vi "SetOverVoltProtLimit.vi"(8 "error in (no error)":errorcluster, 9 "Voltage":dbl, 11 "VISA resource name":refnum<visa-resource-name>) -> (0 "error out":errorcluster, 3 "VISA resource name out":refnum<visa-resource-name>)   [LabVIEW 2019, in "9103Series.lvlib"]
doc: "Set Over Voltage Protection Limit\n\nVoltage: Voltage limit value.\nVoltage Range: 9103 - 42.5, 9104 - 82.5"
uses:
  <instrlib>/9103Series/9103Series.lvlib
panel:
  out "ok?":string
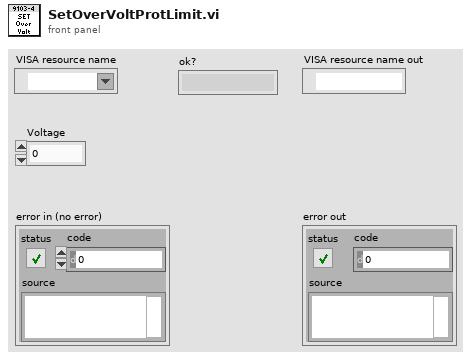
[diagram p1: front panel]
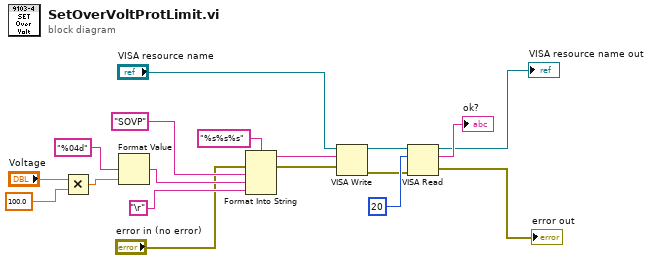
[diagram p0: block diagram]
diagram:
  n1 = Multiply(x="Voltage", y=100.0) -> (x*y=w15:dbl)
  n2 = Format Value(format string="%04d", value (0)=w15) -> (output string=w5:string)  [unwired: 1 in]
  n3 = Format Into String(format string="%s%s%s", error in="error in (no error)", "SOVP" ("string"), w5, "\r") -> (resulting string=w1:string, error out=w2:errorcluster)  [unwired: 1 in]
  n4 = VISA Write(VISA resource name="VISA resource name", write buffer=w1, error in (no error)=w2) -> (VISA resource name out=w9:refnum<visa-resource-name>, error out=w8:errorcluster)  [unwired: 1 out]
  n5 = VISA Read(VISA resource name=w9, byte count=u32 20, error in (no error)=w8) -> (VISA resource name out=→"VISA resource name out":refnum<visa-resource-name>, read buffer=→"ok?":string, error out=→"error out":errorcluster)  [unwired: 1 out]
